vi "SPC_read_rates.vi"(8 "Error In":errorcluster, 10 "Module No":i16 min=0 max=7 step=1, 11 "DLL Path":path) -> (0 "Error Out":errorcluster, 2 "Module No":i16, 3 "DLL Path":path, 4 "SPC_RatesCluster":T1={"Sync"=1728.0, "CFD"=1728.0, "TAC"=848.0, "ADC"=144.0} {"Sync" scale=0.0..6000000.0; "ADC" scale=0.0..1000000.0; "TAC" scale=0.0..1000000.0; "CFD" scale=0.0..1000000.0})   [LabVIEW 2017]
doc: "The procedure reads the rate counters for the SPC module ‘mod_no’, calculates the rate values and writes the results to the ‘rates’ structure.\nThe procedure can be called at any time after an initial call to the SPC_clear_rates function. If the rate values are ready (after 1sec of integration time), the procedure fills ‘rates’, starts a new integration cycle and returns 0, otherwise it returns error -30 -SPC_RATES_NOT_RDY and returns last rates.\nIntegration time of rate values is equal 1sec, but for SPC-13x/830/930/15x/160 modules can have also other values according to the parameter RATE_COUNT_TIME (1.0s, 250ms, 100ms, 50ms are possible).\nTo get correct results the SPC_clear_rates function must be called before the first call of \"SPC_read_rates\". As a default value the parameter \"rate count time\" is set to one second. To change that, please use the \"Set Parameter\" function with the keyword \"rate count time\".\n\n<b>Note:</b> This VI is set to execute as preallocated clone to improve performance when run in parallel loops for multi module setups.\n\ninfo@becker-hickl.com"
uses:
  SPC_Controls/SPC_RatesCluster.ctl
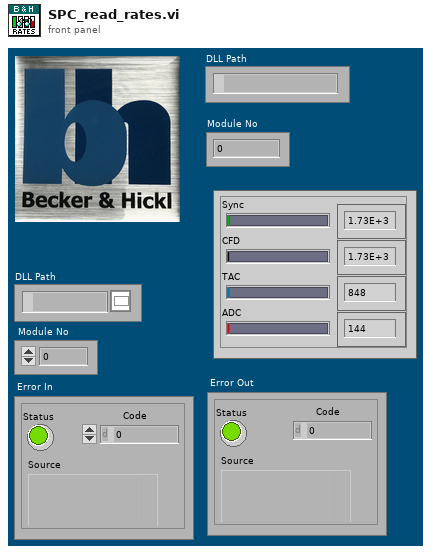
[diagram p1: front panel]
types:
  T1 = typedef "SPC_RatesCluster.ctl" = cluster{"Sync":sgl, "CFD":sgl, "TAC":sgl, "ADC":sgl}
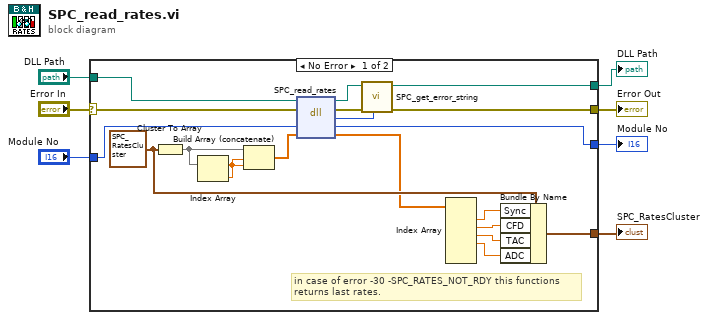
[diagram p0: block diagram]
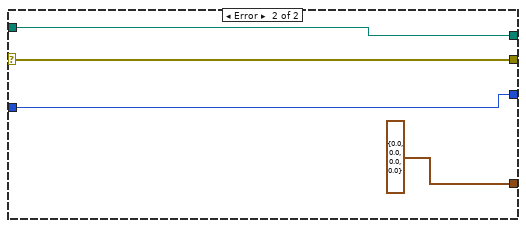
[diagram p2: hidden frame]
diagram:
  n1 = case shown="No Error" "Error In" {
    selector: "Error In" -> [w15 w29]
    tunnel: "DLL Path" -> [w26 w30]
    tunnel: [w20 w30] -> w6
    tunnel: [w17 w29] -> w4
    tunnel: "Module No" -> [w25 w28]
    tunnel: [w24 w28] -> w2
    tunnel: [w16 T1 {"Sync"=0.0, "CFD"=0.0, "TAC"=0.0, "ADC"=0.0} ("CFD TAC ADC Cluster 2")] -> w1
    frame No Error {
      w19 = T1 {"Sync"=1728.0, "CFD"=2909091.0, "TAC"=1939393.4, "ADC"=1424242.4} ("CFD TAC ADC Cluster 2")
      # "in case of error -30 -SPC_RATES_NOT_RDY this functions\nreturns last rates."
      n2 = Cluster To Array(cluster=w19) -> (array=w9:sgl[])
      n3 = Index Array(array=w9) -> (element=w8:sgl)  [unwired: 1 in]
      n4 = Build Array (concatenate)(w9, w8, w8) -> (w10:sgl[])
      n5 = dll-call lib="D:/spcm/lib/lab_view/lv10.0/spcm32.dll" fn="SPC_read_rates"(path in=w26, error in=w15, "mod_no"=w25, "RatesCluster"=w10) -> (path out=w21:path, error out=w22:errorcluster, "return type"=w23:i16, "mod_no"=w24:i16, "RatesCluster"=w18:sgl[])  [unwired: 1 in]
      n6 = call "SPC_get_error_string.vi"("ErrorID"=w23, "Error In"=w22, "DLL Path"=w21) -> ("Error Out"=w17:errorcluster, "DLL Path"=w20:path)  [unwired: 6 in, 1 out]
      n7 = Index Array(array=w18) -> (element #1=w14:sgl, element #2=w13:sgl, element #3=w12:sgl, element #4=w11:sgl)  [unwired: 6 in, 2 out]
      n8 = Bundle By Name(cluster=w19, "Sync"=w14, "CFD"=w13, "TAC"=w12, "ADC"=w11) -> (w16:T1)
    }
    frame Error {
    }
  }
  "DLL Path" <- w6
  "Error Out" <- w4
  "Module No" <- w2
  "SPC_RatesCluster" <- w1
